vi "STED_off_flyback.vi"() -> ()   [LabVIEW 2016]
uses:
  <vilib>/Platform/TimedLoop/XDataNode/timing_clust.ctl
  <vilib>/Platform/TimedLoop/XDataNode/nitl_modes.ctl
  <vilib>/Platform/TimedLoop/XDataNode/wakeup.ctl
  <vilib>/rvi/Emulation/niFpgaGetClockAttributes.vi
  <vilib>/rvi/Emulation/niFpgaSctlEmulationGetInTimedLoop.vi
  <vilib>/rvi/Emulation/niFpgaEmulationReportErrorSimple.vi
  <vilib>/rvi/eio/common/nirviEmuTemplateMethod_errors.vi
  <vilib>/rvi/Emulation/niFpgaCriticalErrorInLSC.vi
  <vilib>/eio/EIONode/EIONode.xnode
  <vilib>/Platform/TimedLoop/XDataNode/XDataNode.xnode
  <vilib>/Platform/TimedLoop/XDataNode/XDNodeRunTimeDep.lvlib
panel:
  in  "turn off STED after":i64
  in  "stop 2":bool
  in  "AOM Volts":u16[](array[numeric])=[0, 82, 164, 246]
  in  "stop 1":bool
  # "nominal 12 bit ADC volts"
  # ".1=82\n.2=164\n.3=246"
  # "Turn off STED laser after this many 12.5 ns cycles without a new pixel clock trigger event\n\n320= one 4 us pixel dwell time in clock cycles\n800 = one 10 us pixel dwell time in clock cycles."
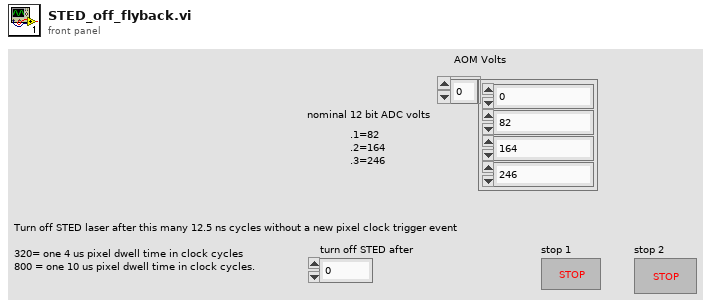
[diagram p1: front panel]
types:
  T1 = typedef "XDNodeRunTimeDep.lvlib/timing_clust.ctl" = cluster{"Expected End [f-1]":u64, "Actual End [f-1]":u64, "Finished Late? [f-1]":bool, "Expected End [i-1]":u64, "Actual End [i-1]":u64, "Finished Late? [i-1]":bool, "Expected Start [i]":u64, "Actual Start [i]":u64, "Expected Start [f]":u64, "Actual Start [f]":u64, "Source Name":string, "Structure Name":string, "Period":i64, "Deadline":i64, "Offset":i64, "Start":i64, "Priority":i32, "Timeout":i32, "Mode":T2, "Wakeup Reason":T3, "Error":errorcluster, "Source Type":string, "Secondary Source Type":string, "Global End Time":u64, "Global Start Time":u64, "Frame Duration":u64, "Iteration Duration":u64, "Assigned CPU":i32, "I/O Scan Engine Mode":u32}
  T2 = typedef "XDNodeRunTimeDep.lvlib/nitl_modes.ctl" = enum32{"No Change", "Process missed periods, maintain original phase", "Discard missed periods, maintain original phase", "Process missed periods, ignore original phase", "Discard missed periods, ignore original phase"}
  T3 = typedef "XDNodeRunTimeDep.lvlib/wakeup.ctl" = enum32{"Normal", "Aborted", "Asynchronous wakeup", "Timing source error", "Timed loop error", "Timeout"}
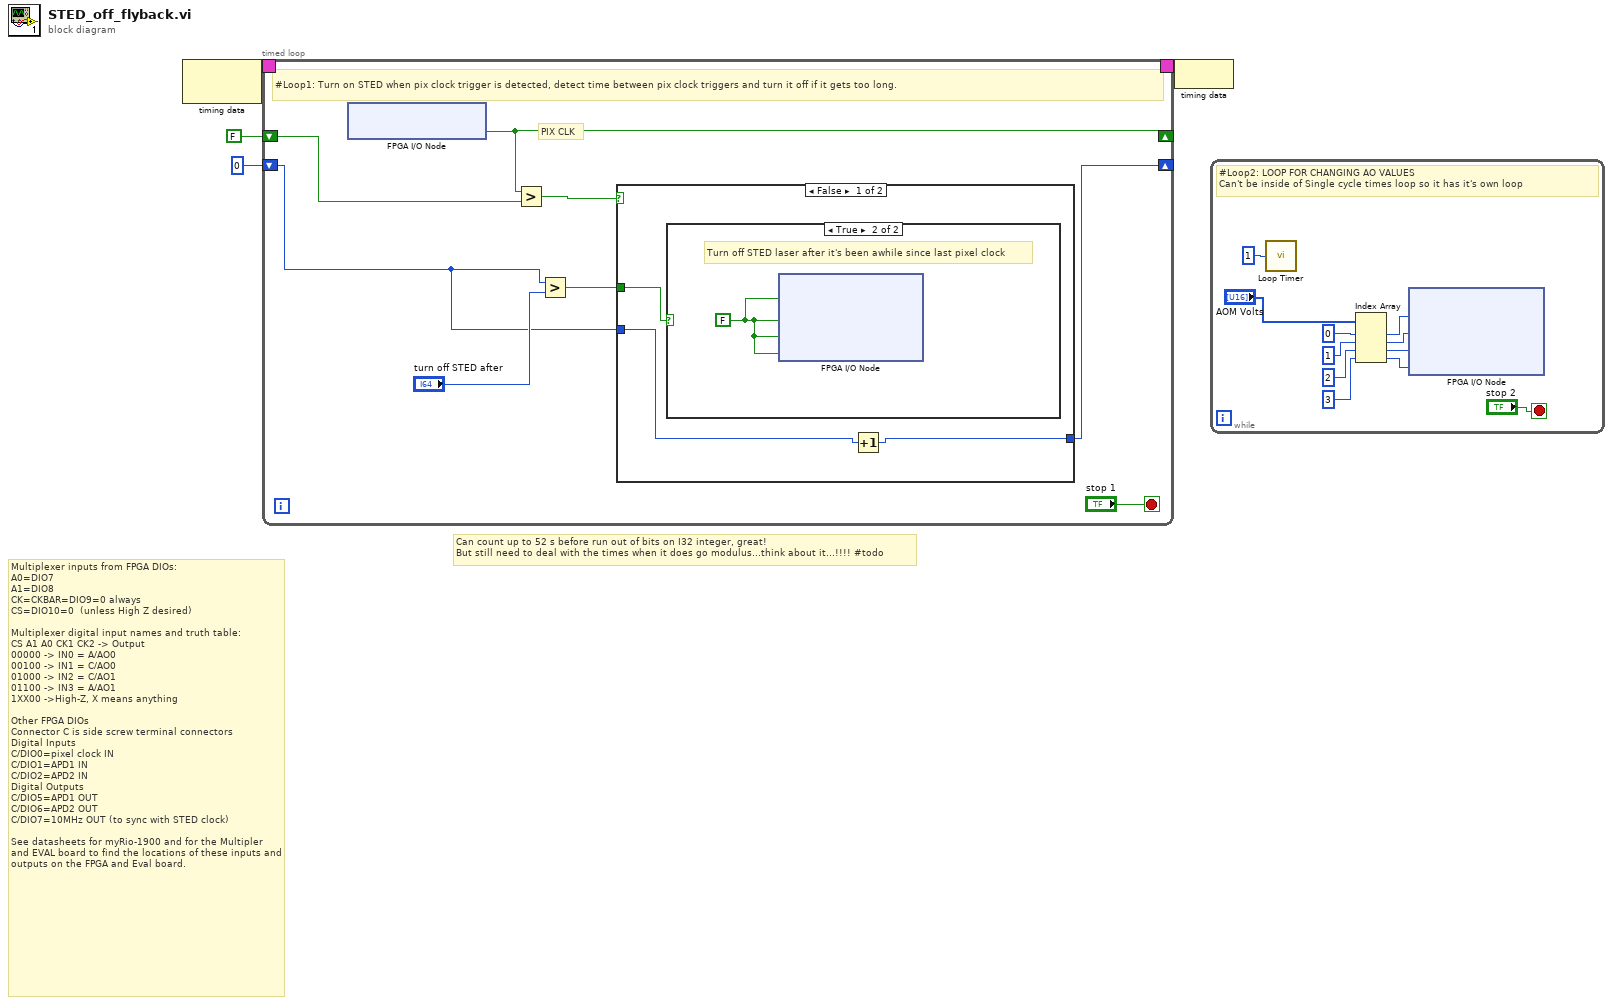
[diagram p0: block diagram]
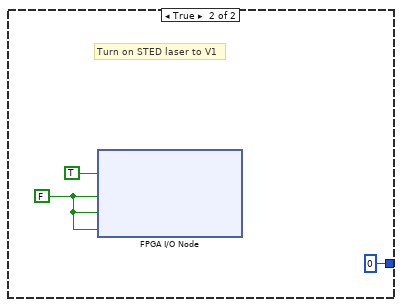
[diagram p3: hidden frame]
diagram:
  # "Can count up to 52 s before run out of bits on I32 integer, great!\nBut still need to deal with the times when it does go modulus...think about it...!!!! #todo"
  # "Multiplexer inputs from FPGA DIOs:\nA0=DIO7\nA1=DIO8\nCK=CKBAR=DIO9=0 always\nCS=DIO10=0  (unless High Z desired)\n\nMultiplexer digital input names and truth table:\nCS A1 A0 CK1 CK2 -> Output\n00000 -> IN0 = A/AO0\n00100 -> IN1 = C/AO0\n01000 -> IN2 = C/AO1\n01100 -> IN3 = A/AO1\n1XX00 ->High-Z, X means anything\n\nOther FPGA DIOs\nConnector C is side screw terminal connectors\nDigital Inputs\nC/DIO0=pixel clock IN\nC/DIO1=APD1 IN\nC/DIO2=APD2 IN\nDigital Outputs\nC/DIO5=APD1 OUT\nC/DIO6=APD2 OUT\nC/DIO7=10MHz OUT (to sync with STED clock)\n\nSee datasheets for myRio-1900 and for the Multipler and EVAL board to find the locations of these inputs and outputs on the FPGA and Eval board."
  n1 = node-c288() -> (w4:T1)  [unwired: 1 in]
  n2 = timed-loop {
    timing: w4 -> [_]
    timing-out: [_] -> w3
    shift-right: [w10] -> _
    shift-left: FALSE -> [w12]
    shift-right: [w8] -> _
    shift-left: i64 0 -> [w5]
    stop <- "stop 1" stop-if-true
    # "PIX CLK"
    # "#Loop1: Turn on STED when pix clock trigger is detected, detect time between pix clock triggers and turn it off if it gets too long."
    n3 = xnode "FPGA I/O Node"() -> ("ConnectorC/DIO0"=w10:bool)  [unwired: 1 in, 1 out]
    n4 = Greater?(x=w10, y=w12) -> (0:w9:bool)
    n5 = Greater?(x=w5, y="turn off STED after") -> (0:w6:bool)
    n6 = case shown="False" w9 {
      tunnel: [w13 i64 0] -> w8
      tunnel: w5 -> [w14 _]
      tunnel: w6 -> [w15 _]
      frame False {
        n7 = case shown="True" w15 {
          frame False {
          }
          frame True {
            w16 = FALSE ("ConnectorA/DIO8")
            # "Turn off STED laser after it's been awhile since last pixel clock"
            n8 = xnode "FPGA I/O Node"("ConnectorA/DIO7"=w16, "ConnectorA/DIO8"=w16, "ConnectorA/DIO9"=w16, "ConnectorA/DIO10"=w16) -> ()  [unwired: 4 in, 4 out]
          }
        }
        n9 = Increment(x=w14) -> (x+1=w13:i64)
      }
      frame True {
        w18 = FALSE ("ConnectorA/DIO8")
        # "Turn on STED laser to V1"
        n10 = xnode "FPGA I/O Node"("ConnectorA/DIO7"=TRUE, "ConnectorA/DIO8"=w18, "ConnectorA/DIO9"=w18, "ConnectorA/DIO10"=w18) -> ()  [unwired: 4 in, 4 out]
      }
    }
  }
  n11 = node-c288(w3) -> ()
  n12 = while {
    stop <- "stop 2" stop-if-true
    # "#Loop2: LOOP FOR CHANGING AO VALUES\nCan't be inside of Single cycle times loop so it has it's own loop"
    n13 = call "Loop Timer"("Count(mSec)"=u32 1) -> ()  [unwired: 1 out]
    n14 = Index Array(array="AOM Volts", index #1=0 ("index"), index #2=1 ("index"), index #3=2 ("index"), index #4=3 ("index")) -> (element #1=w28:u16, element #2=w24:u16, element #3=w23:u16, element #4=w25:u16)
    n15 = xnode "FPGA I/O Node"("ConnectorA/AO0"=w28, "ConnectorC/AO0"=w24, "ConnectorC/AO1"=w23, "ConnectorA/AO1"=w25) -> ()  [unwired: 4 in, 4 out]
  }
